vi "Read List Data.vi"(6 "Sequence Repeat Count":i32[](array[numeric]), 8 "error in":errorcluster, 10 "List Number":i32, 11 "VISA resource name":refnum<visa-resource-name>) -> (0 "error out":errorcluster, 1 "List Repeat":i32=1 min=1 max=65535 step=1, 2 "Sequence Repeat Count Out":i32[](array[numeric]), 3 "VISA resource name out":refnum<visa-resource-name>, 4 "Linked Sequences":bool[](array[boolean]), 5 "List Power Limit":dbl)   [LabVIEW 2022 SP3]
uses:
  <instrlib>/BK Precision 911X Series/BK Precision 911X Series.lvlib
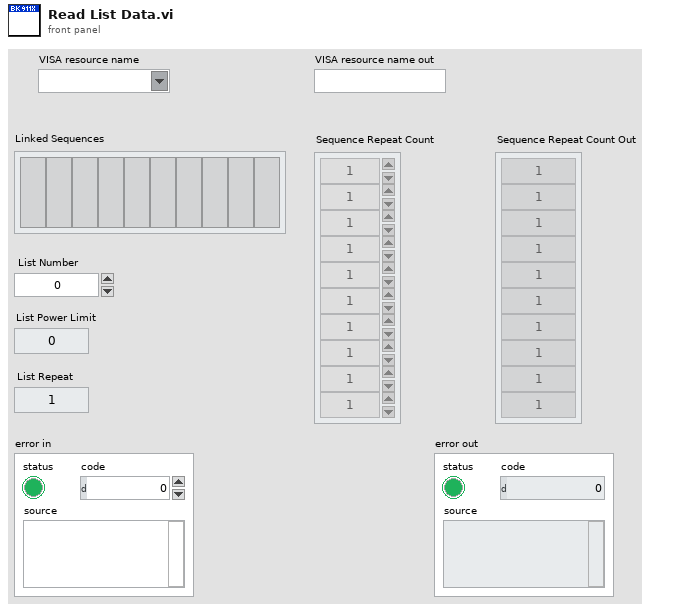
[diagram p1: front panel]
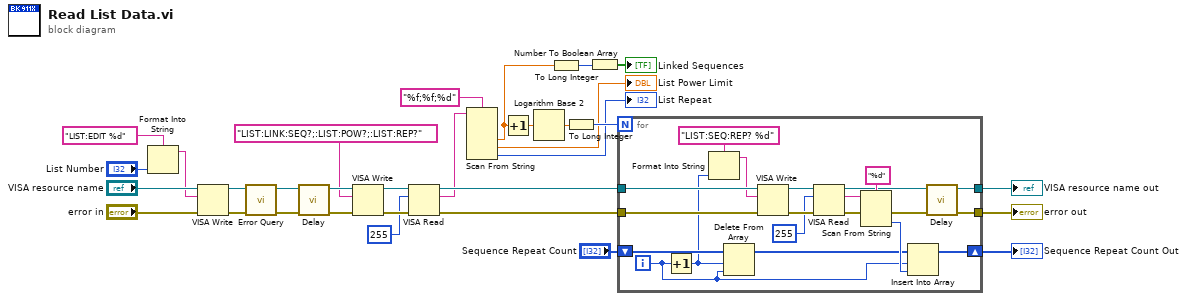
[diagram p0: block diagram]
diagram:
  n1 = Format Into String(format string="LIST:EDIT %d" ("write buffer"), "List Number") -> (resulting string=w26:string)  [unwired: 2 in, 1 out]
  n2 = VISA Write(VISA resource name="VISA resource name", write buffer=w26, error in (no error)="error in") -> (VISA resource name out=w21:refnum<visa-resource-name>, error out=w20:errorcluster)  [unwired: 1 out]
  n3 = call <instrlib>:"Error Query.vi"("error in (no error)"=w20, "VISA resource name"=w21) -> ("error out"=w29:errorcluster, "VISA resource name out"=w30:refnum<visa-resource-name>)  [unwired: 6 in, 2 out]
  n4 = call "Delay.vi"("error in (no error)"=w29, "VISA resource name"=w30) -> ("error out"=w18:errorcluster, "VISA resource name out"=w19:refnum<visa-resource-name>)  [unwired: 8 in]
  n5 = VISA Write(VISA resource name=w19, write buffer="LIST:LINK:SEQ?;:LIST:POW?;:LIST:REP?", error in (no error)=w18) -> (VISA resource name out=w24:refnum<visa-resource-name>, error out=w23:errorcluster)  [unwired: 1 out]
  n6 = VISA Read(VISA resource name=w24, byte count=u32 255, error in (no error)=w23) -> (VISA resource name out=w16:refnum<visa-resource-name>, read buffer=w14:string, error out=w15:errorcluster)  [unwired: 1 out]
  n7 = Scan From String(format string="%f;%f;%d", input string=w14) -> (output 1=w5:dbl, output 2=→"List Power Limit":dbl, output 3=→"List Repeat":i32)  [unwired: 5 in, 3 out]
  n8 = Increment(x=w5) -> (x+1=w7:dbl)
  n9 = Logarithm Base 2(1:w7) -> (0:w4:dbl)
  n10 = To Long Integer(number=w5) -> (32bit integer=w6:i32)
  n11 = To Long Integer(number=w4) -> (32bit integer=w3:i32)
  n12 = Number To Boolean Array(number=w6) -> (Boolean array=→"Linked Sequences":bool[])
  n13 = for {
    N: w3 -> [_]
    tunnel: w16 -> [w47]
    tunnel: w15 -> [w46]
    tunnel: [w39] -> w11
    tunnel: [w38] -> w10
    shift-right: [w36] -> w8
    shift-left: "Sequence Repeat Count" -> [w35]
    i -> [w33]
    n14 = Increment(x=w33) -> (x+1=w32:i32)
    n15 = Format Into String(format string="LIST:SEQ:REP? %d" ("write buffer"), w32) -> (resulting string=w45:string)  [unwired: 2 in, 1 out]
    n16 = Delete From Array(array=w35, length=w32, index=w33) -> (array with subset deleted=w34:i32[])  [unwired: 1 out]
    n17 = VISA Write(VISA resource name=w47, write buffer=w45, error in (no error)=w46) -> (VISA resource name out=w48:refnum<visa-resource-name>, error out=w50:errorcluster)  [unwired: 1 out]
    n18 = VISA Read(VISA resource name=w48, byte count=u32 255, error in (no error)=w50) -> (VISA resource name out=w40:refnum<visa-resource-name>, read buffer=w43:string, error out=w41:errorcluster)  [unwired: 1 out]
    n19 = Scan From String(format string="%d", input string=w43) -> (output 1=w37:i32)  [unwired: 3 in, 3 out]
    n20 = Insert Into Array(array=w34, index=w33, new element=w37) -> (w36:i32[])
    n21 = call "Delay.vi"("error in (no error)"=w41, "VISA resource name"=w40) -> ("error out"=w39:errorcluster, "VISA resource name out"=w38:refnum<visa-resource-name>)  [unwired: 8 in]
  }
  "VISA resource name out" <- w10
  "error out" <- w11
  "Sequence Repeat Count Out" <- w8
